vi "Settings Dialog.vi"(8 "error in (no error)":errorcluster, 11 "Settings in":T3={"Logging Configuration"={"Log File Base Path"=path "", "Max Samples"=0, "File Refnum"=refnum, "Log Piezo"=FALSE, "Piezo File Refnum"=refnum, "Log Capacitive"=FALSE, "Cap File Refnum"=refnum, "Filename"="", "Path where to save"=path ""}, "Piezo Config"={"Piezo Serial Number"=41848555, "MG17Piezo"=refnum, "Setpoint (um)"=0.0}, "Capacitive Config"={"IP Address"="192.168.168.57", "Handle"=0, "Refresh Time (ms)"=0.0}, "Hardware Config"={"Data Source"=0, "Counter Configuration"={"DAQmx Task"="", "Counter(s)"="Dev2/ctr0", "samples per readout"=100}, "ADC Configuration"={"DAQmx Task"="", "Channel(s)"="Dev2/ctr0", "samples per readout"=100, "Sample Rate (s/s)"=100, "Max Voltage"=100.0, "Min Voltage"=100.0}}} {"Hardware Config"."Data Source" items=["Counter", "ADC"]}) -> (0 "error out":errorcluster, 1 "Cancelled?":bool=TRUE, 2 "UI Refresh Needed?":bool, 3 "Settings out":T3={"Logging Configuration"={"Log File Base Path"=path "", "Max Samples"=0, "File Refnum"=refnum, "Log Piezo"=FALSE, "Piezo File Refnum"=refnum, "Log Capacitive"=FALSE, "Cap File Refnum"=refnum, "Filename"="", "Path where to save"=path ""}, "Piezo Config"={"Piezo Serial Number"=41848555, "MG17Piezo"=refnum, "Setpoint (um)"=0.0}, "Capacitive Config"={"IP Address"="192.168.168.57", "Handle"=0, "Refresh Time (ms)"=0.0}, "Hardware Config"={"Data Source"=0, "Counter Configuration"={"DAQmx Task"="", "Counter(s)"="Dev2/ctr0", "samples per readout"=100}, "ADC Configuration"={"DAQmx Task"="", "Channel(s)"="Dev2/ctr0", "samples per readout"=100, "Sample Rate (s/s)"=100, "Max Voltage"=100.0, "Min Voltage"=100.0}}} {"Hardware Config"."Data Source" items=["Counter", "ADC"]})   [LabVIEW 2013, in "Settings.lvlib"]
doc: "Dialog for selecting user specified settings."
uses:
  Settings.lvlib
  Settings.ctl
  Logging/Logging Configuration.ctl
  Piezo/Hardware Configuration.ctl
  Capacitive/Hardware Configuration.ctl
  Acquisition/Hardware Configuration.ctl
  Acquisition/Counter Configuration.ctl
  ADC/ADC Configuration.ctl
  <vilib>/Utility/xml.llb/Write to XML File(string).vi
  Acquisition/Acquisition.lvlib
  Logging/Logging.lvlib
  Piezo/Piezo.lvlib
  Capacitive/Capacitive.lvlib
panel:
  in  "Log Capacitive?":bool
  in  "ADC Configuration":T1={"Channel(s)"="Dev2/ctr0", "samples per readout"=100, "Sample Rate"=100, "Vmax"=100.0}
  in  "Counter Configuration":T2={"Counter(s)"="Dev2/ctr0", "samples per readout"=100}
  in  "Data Source":u16(ring) items=["Counter", "ADC"]
  in  "Refresh Time (ms)":dbl
  in  "IP Address":string
  in  "Log Piezo?":bool
  in  "Max Samples":u32
  in  "Log File Path":path
  in  "Cancel Button":bool
  in  "OK Button":bool
  # "Acquisition"
  # "Non visible portion of dialog (needed for connector pane)."
  # "Logging"
  # "Capacitive Sensor"
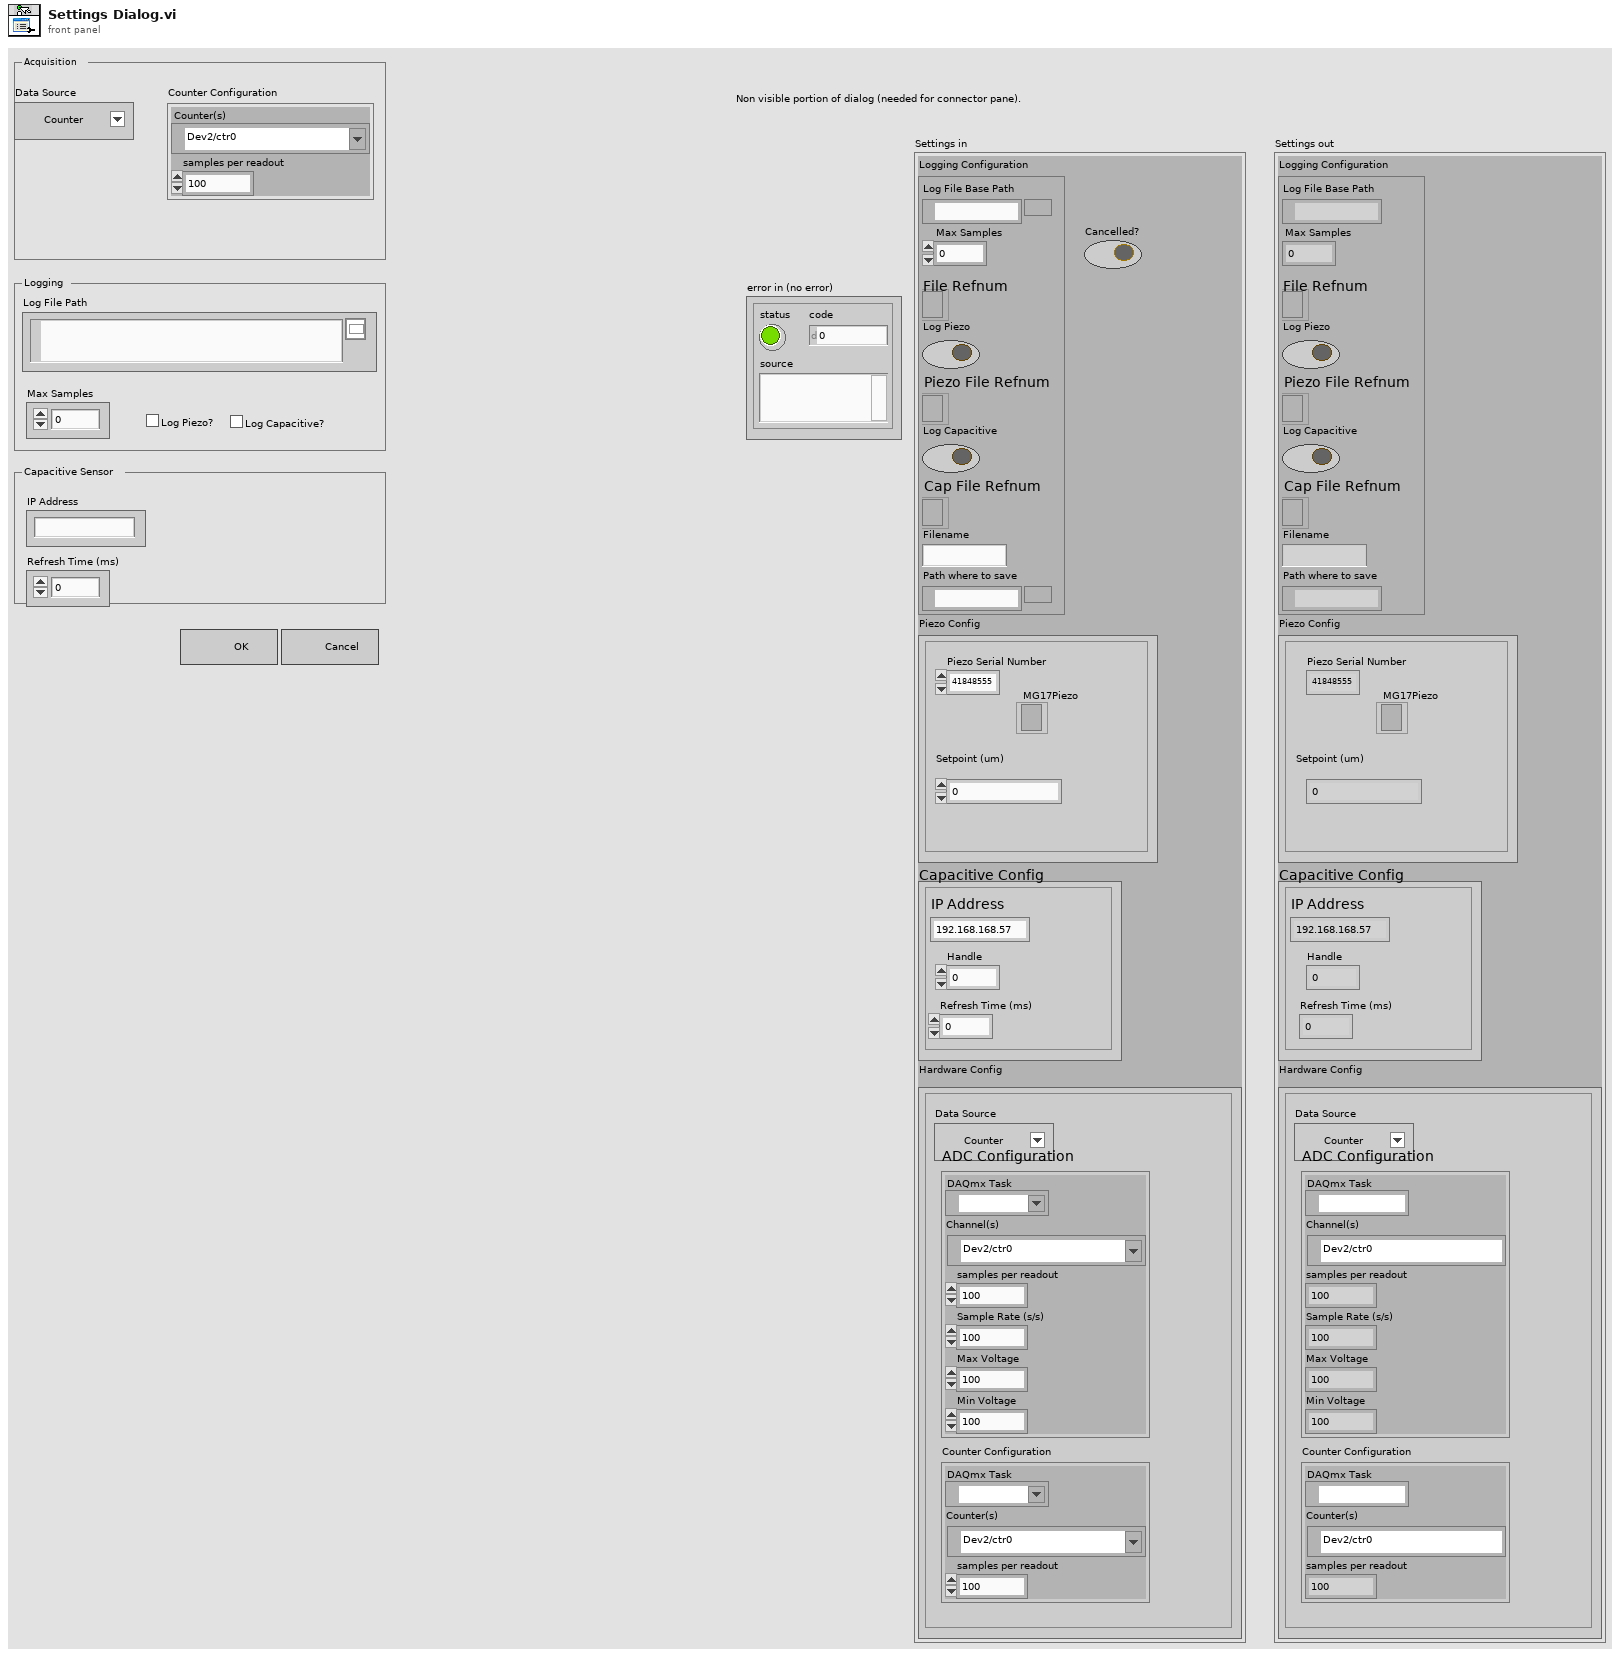
[diagram p1: front panel]
types:
  T1 = cluster{"Channel(s)":tag, "samples per readout":i32, "Sample Rate":i32, "Vmax":dbl}
  T2 = cluster{"Counter(s)":tag, "samples per readout":i32}
  T3 = typedef "Settings.lvlib/Settings.ctl" = cluster{"Logging Configuration":T4, "Piezo Config":T5, "Capacitive Config":T6, "Hardware Config":T7}
  T4 = typedef "Logging.lvlib/Logging Configuration.ctl" = cluster{"Log File Base Path":path, "Max Samples":u32, "File Refnum":refnum<file>, "Log Piezo":bool, "Piezo File Refnum":refnum<file>, "Log Capacitive":bool, "Cap File Refnum":refnum<file>, "Filename":string, "Path where to save":path}
  T5 = typedef "Piezo.lvlib/Hardware Configuration.ctl" = cluster{"Piezo Serial Number":i32, "MG17Piezo":refnum<k7>, "Setpoint (um)":sgl}
  T6 = typedef "Capacitive.lvlib/Hardware Configuration.ctl" = cluster{"IP Address":string, "Handle":u32, "Refresh Time (ms)":dbl}
  T7 = typedef "Acquisition.lvlib/Hardware Configuration.ctl" = cluster{"Data Source":u16, "Counter Configuration":T8, "ADC Configuration":T9}
  T8 = typedef "Acquisition.lvlib/Counter Configuration.ctl" = cluster{"DAQmx Task":refnum<k21>, "Counter(s)":tag, "samples per readout":i32}
  T9 = typedef "Acquisition.lvlib/ADC Configuration.ctl" = cluster{"DAQmx Task":refnum<k21>, "Channel(s)":tag, "samples per readout":i32, "Sample Rate (s/s)":i32, "Max Voltage":dbl, "Min Voltage":dbl}
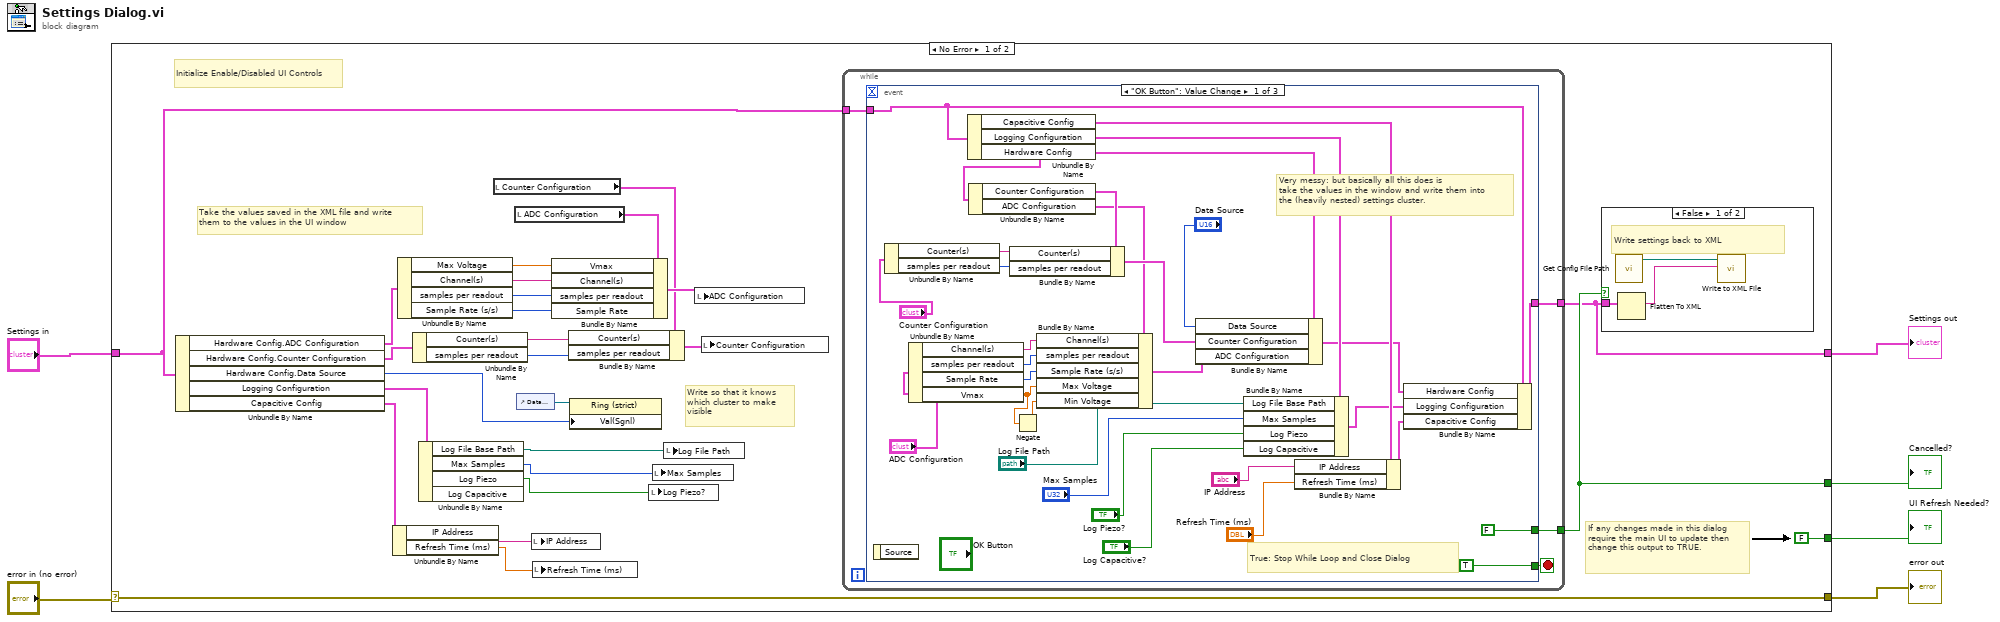
[diagram p0: block diagram]
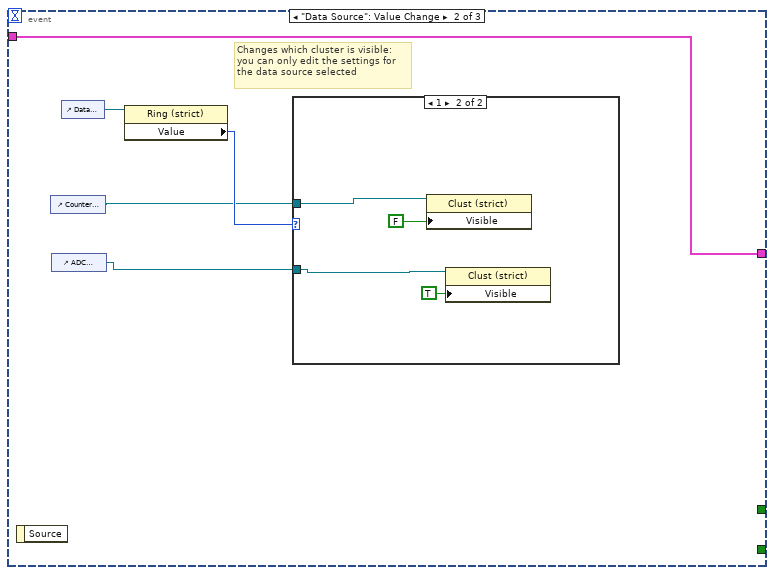
[diagram p2: hidden frame]
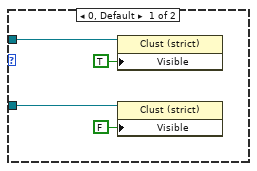
[diagram p3: hidden frame]
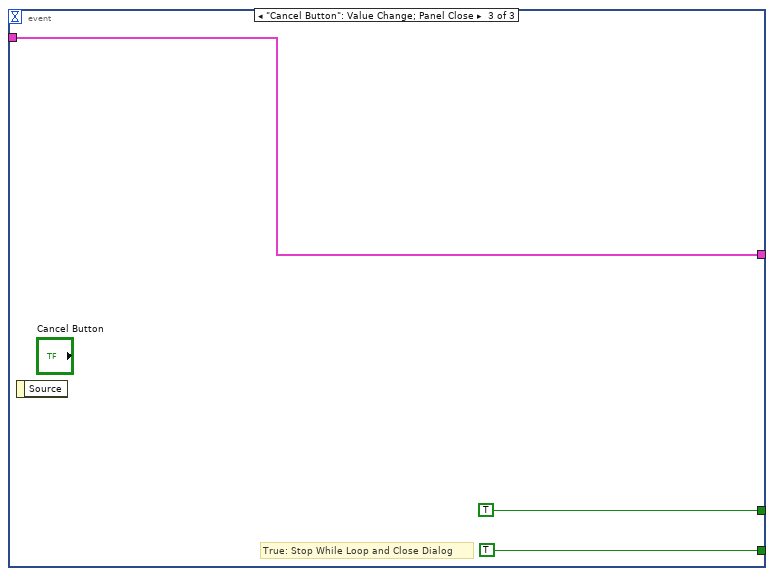
[diagram p4: hidden frame]
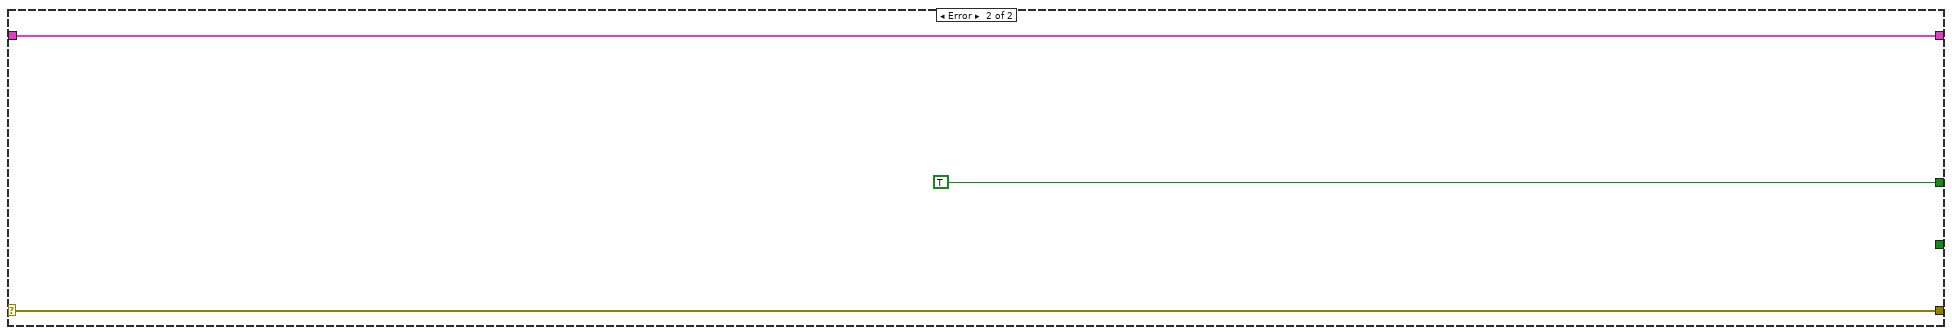
[diagram p6: hidden frame]
diagram:
  n1 = case shown="No Error" "error in (no error)" {
    selector: "error in (no error)" -> [w32 w88]
    tunnel: [w32 w88] -> w6
    tunnel: "Settings in" -> [w28 w87]
    tunnel: [w29 w87] -> w4
    tunnel: [FALSE ("UI Refresh Needed?") _] -> w3
    tunnel: [w30 TRUE ("UI Refresh Needed?")] -> w2
    frame No Error {
      # "Write so that it knows\nwhich cluster to make \nvisible"
      # "Take the values saved in the XML file and write\nthem to the values in the UI window"
      # "Initialize Enable/Disabled UI Controls"
      # "If any changes made in this dialog require the main UI to update then change this output to TRUE."
      n2 = Unbundle By Name(w28) -> ("Hardware Config.ADC Configuration"=w14:T9, "Hardware Config.Counter Configuration"=w18:T8, "Hardware Config.Data Source"=w19:u16, "Logging Configuration"=w24:T4, "Capacitive Config"=w27:T6)
      n3 = Unbundle By Name(w27) -> ("IP Address"=w26:string, "Refresh Time (ms)"=w25:dbl)
      n4 = Unbundle By Name(w14) -> ("Max Voltage"=w7:dbl, "Channel(s)"=w13:tag, "samples per readout"=w12:i32, "Sample Rate (s/s)"=w11:i32)
      n5 = Unbundle By Name(w18) -> ("Counter(s)"=w17:tag, "samples per readout"=w16:i32)
      n6 = Unbundle By Name(w24) -> ("Log File Base Path"=w21:path, "Max Samples"=w22:u32, "Log Piezo"=w23:bool)  [unwired: 1 out]
      n7 = local read "Counter Configuration"() -> (w8:T2)
      n8 = local read "ADC Configuration"() -> (w9:T1)
      n9 = control-ref of="Data Source"() -> (w20:refnum<vi>)
      n10 = local write "IP Address"(w26) -> ()
      n11 = local write "Refresh Time (ms)"(w25) -> ()
      n12 = Bundle By Name(cluster=w9, "Vmax"=w7, "Channel(s)"=w13, "samples per readout"=w12, "Sample Rate"=w11) -> (w10:T1)
      n13 = Bundle By Name(cluster=w8, "Counter(s)"=w17, "samples per readout"=w16) -> (w15:T2)
      n14 = property class="Ring (strict)"(reference=w20, "Val(Sgnl)"=w19) -> ()  [unwired: 1 in, 2 out]
      n15 = local write "Log Piezo?"(w23) -> ()
      n16 = local write "Max Samples"(w22) -> ()
      n17 = local write "Log File Path"(w21) -> ()
      n18 = local write "ADC Configuration"(w10) -> ()
      n19 = local write "Counter Configuration"(w15) -> ()
      n20 = while {
        tunnel: [w36] -> w30
        tunnel: [w35] -> w29
        tunnel: w28 -> [w34]
        stop <- w33 stop-if-true
        n21 = event shown="[0] \"OK Button\": Value Change" {
          selector: _ -> [_ _ _]
          dyn-events: _ -> [_ _ _]
          timeout: _ -> [_ _ _]
          tunnel: [w64 w71 w82] -> w35
          tunnel: w34 -> [w61 w71 w82]
          tunnel: [FALSE ("UI Refresh Needed?") _ TRUE ("UI Refresh Needed?")] -> w36
          tunnel: [TRUE _ TRUE] -> w33
          event "OK Button": Value Change {
            # "Very messy: but basically all this does is\ntake the values in the window and write them into\nthe (heavily nested) settings cluster."
            # "True: Stop While Loop and Close Dialog"
            n22 = event-data() -> ()  [unwired: 1 in, 1 out]
            n23 = Unbundle By Name("Counter Configuration") -> ("Counter(s)"=w48:tag, "samples per readout"=w47:i32)
            n24 = Unbundle By Name("ADC Configuration") -> ("Channel(s)"=w42:tag, "samples per readout"=w43:i32, "Sample Rate"=w44:i32, "Vmax"=w39:dbl)
            n25 = Unbundle By Name(w61) -> ("Capacitive Config"=w60:T6, "Logging Configuration"=w58:T4, "Hardware Config"=w51:T7)
            n26 = Unbundle By Name(w51) -> ("Counter Configuration"=w49:T8, "ADC Configuration"=w45:T9)
            n27 = Bundle By Name(cluster=w49, "Counter(s)"=w48, "samples per readout"=w47) -> (w50:T8)
            n28 = Negate(x=w39) -> (-x=w38:dbl)
            n29 = Bundle By Name(cluster=w45, "Channel(s)"=w42, "samples per readout"=w43, "Sample Rate (s/s)"=w44, "Max Voltage"=w39, "Min Voltage"=w38) -> (w46:T9)
            n30 = Bundle By Name(cluster=w51, "Data Source"="Data Source", "Counter Configuration"=w50, "ADC Configuration"=w46) -> (w53:T7)
            n31 = Bundle By Name(cluster=w58, "Log File Base Path"="Log File Path", "Max Samples"="Max Samples", "Log Piezo"="Log Piezo?", "Log Capacitive"="Log Capacitive?") -> (w54:T4)
            n32 = Bundle By Name(cluster=w60, "IP Address"="IP Address", "Refresh Time (ms)"="Refresh Time (ms)") -> (w63:T6)
            n33 = Bundle By Name(cluster=w61, "Hardware Config"=w53, "Logging Configuration"=w54, "Capacitive Config"=w63) -> (w64:T3)
          }
          event "Data Source": Value Change {
            # "Changes which cluster is visible:\nyou can only edit the settings for\nthe data source selected"
            n34 = event-data() -> ()  [unwired: 1 in, 1 out]
            n35 = control-ref of="Counter Configuration"() -> (w68:refnum<vi>)
            n36 = control-ref of="ADC Configuration"() -> (w67:refnum<vi>)
            n37 = control-ref of="Data Source"() -> (w70:refnum<vi>)
            n38 = property class="Ring (strict)"(reference=w70) -> ("Value"=w69:u16)  [unwired: 1 in, 2 out]
            n39 = case shown="1" w69 {
              tunnel: w68 -> [w75 w77]
              tunnel: w67 -> [w74 w76]
              frame 0, Default {
                n40 = property class="Clust (strict)"(reference=w75, "Visible"=TRUE) -> ()  [unwired: 1 in, 2 out]
                n41 = property class="Clust (strict)"(reference=w74, "Visible"=FALSE) -> ()  [unwired: 1 in, 2 out]
              }
              frame 1 {
                n42 = property class="Clust (strict)"(reference=w77, "Visible"=FALSE) -> ()  [unwired: 1 in, 2 out]
                n43 = property class="Clust (strict)"(reference=w76, "Visible"=TRUE) -> ()  [unwired: 1 in, 2 out]
              }
            }
          }
          event "Cancel Button": Value Change; Panel Close {
            # "True: Stop While Loop and Close Dialog"
            n44 = event-data() -> ()  [unwired: 1 in, 1 out]
          }
        }
      }
      n45 = case shown="False" w30 {
        tunnel: w29 -> [w84 _]
        frame False {
          # "Write settings back to XML"
          n46 = call "Get Config File Path.vi"() -> ("XML File Path"=w85:path)  [unwired: 10 in, 1 out]
          n47 = Flatten To XML(anything=w84) -> (xml string=w83:string)
          n48 = call-poly <vilib>:"Write to XML File.vi"("XML Input"=w83, "XML File Path"=w85) -> ()  [unwired: 7 in, 3 out]
        }
        frame True {
        }
      }
    }
    frame Error {
    }
  }
  "UI Refresh Needed?" <- w3
  "error out" <- w6
  "Settings out" <- w4
  "Cancelled?" <- w2
